vi "Arthur_Q2_VF.vi"() -> ()   [LabVIEW 2019]
uses:
  <vilib>/Waveform/WDTOps.llb/WDT Get Waveform Subset DBL.vi
  <vilib>/measure/matone.llb/Extract Single Tone Information 1 Chan.vi
  <vilib>/measure/NI_MAPro.lvlib
panel:
  out "Numeric 2":dbl
  out "Numeric":dbl
  out "String 2":string="AFUNDAMENTO"
  out "String":string="ELEVA敲O"
  out "Waveform Graph 6":waveform(dbl)(graph)
  out "Waveform Graph 5":waveform(dbl)(graph)
  in  "PATH_2":path=path "C:/lista3.tdms"
  in  "Phase 3":dbl caption="Phase"
  in  "Amplitude 3":dbl=0.5 caption="Amplitude"
  in  "Frequency 3":dbl=40.0 caption="Frequency"
  in  "Phase 2":dbl caption="Phase"
  in  "Amplitude 2":dbl=1.0 caption="Amplitude"
  in  "Frequency 2":dbl=20.0 caption="Frequency"
  in  "Phase":dbl
  in  "Amplitude":dbl=2.0
  in  "Frequency":dbl=10.0
  out "Waveform Graph":dynamicdata(graph)
  # "Phase em graus"
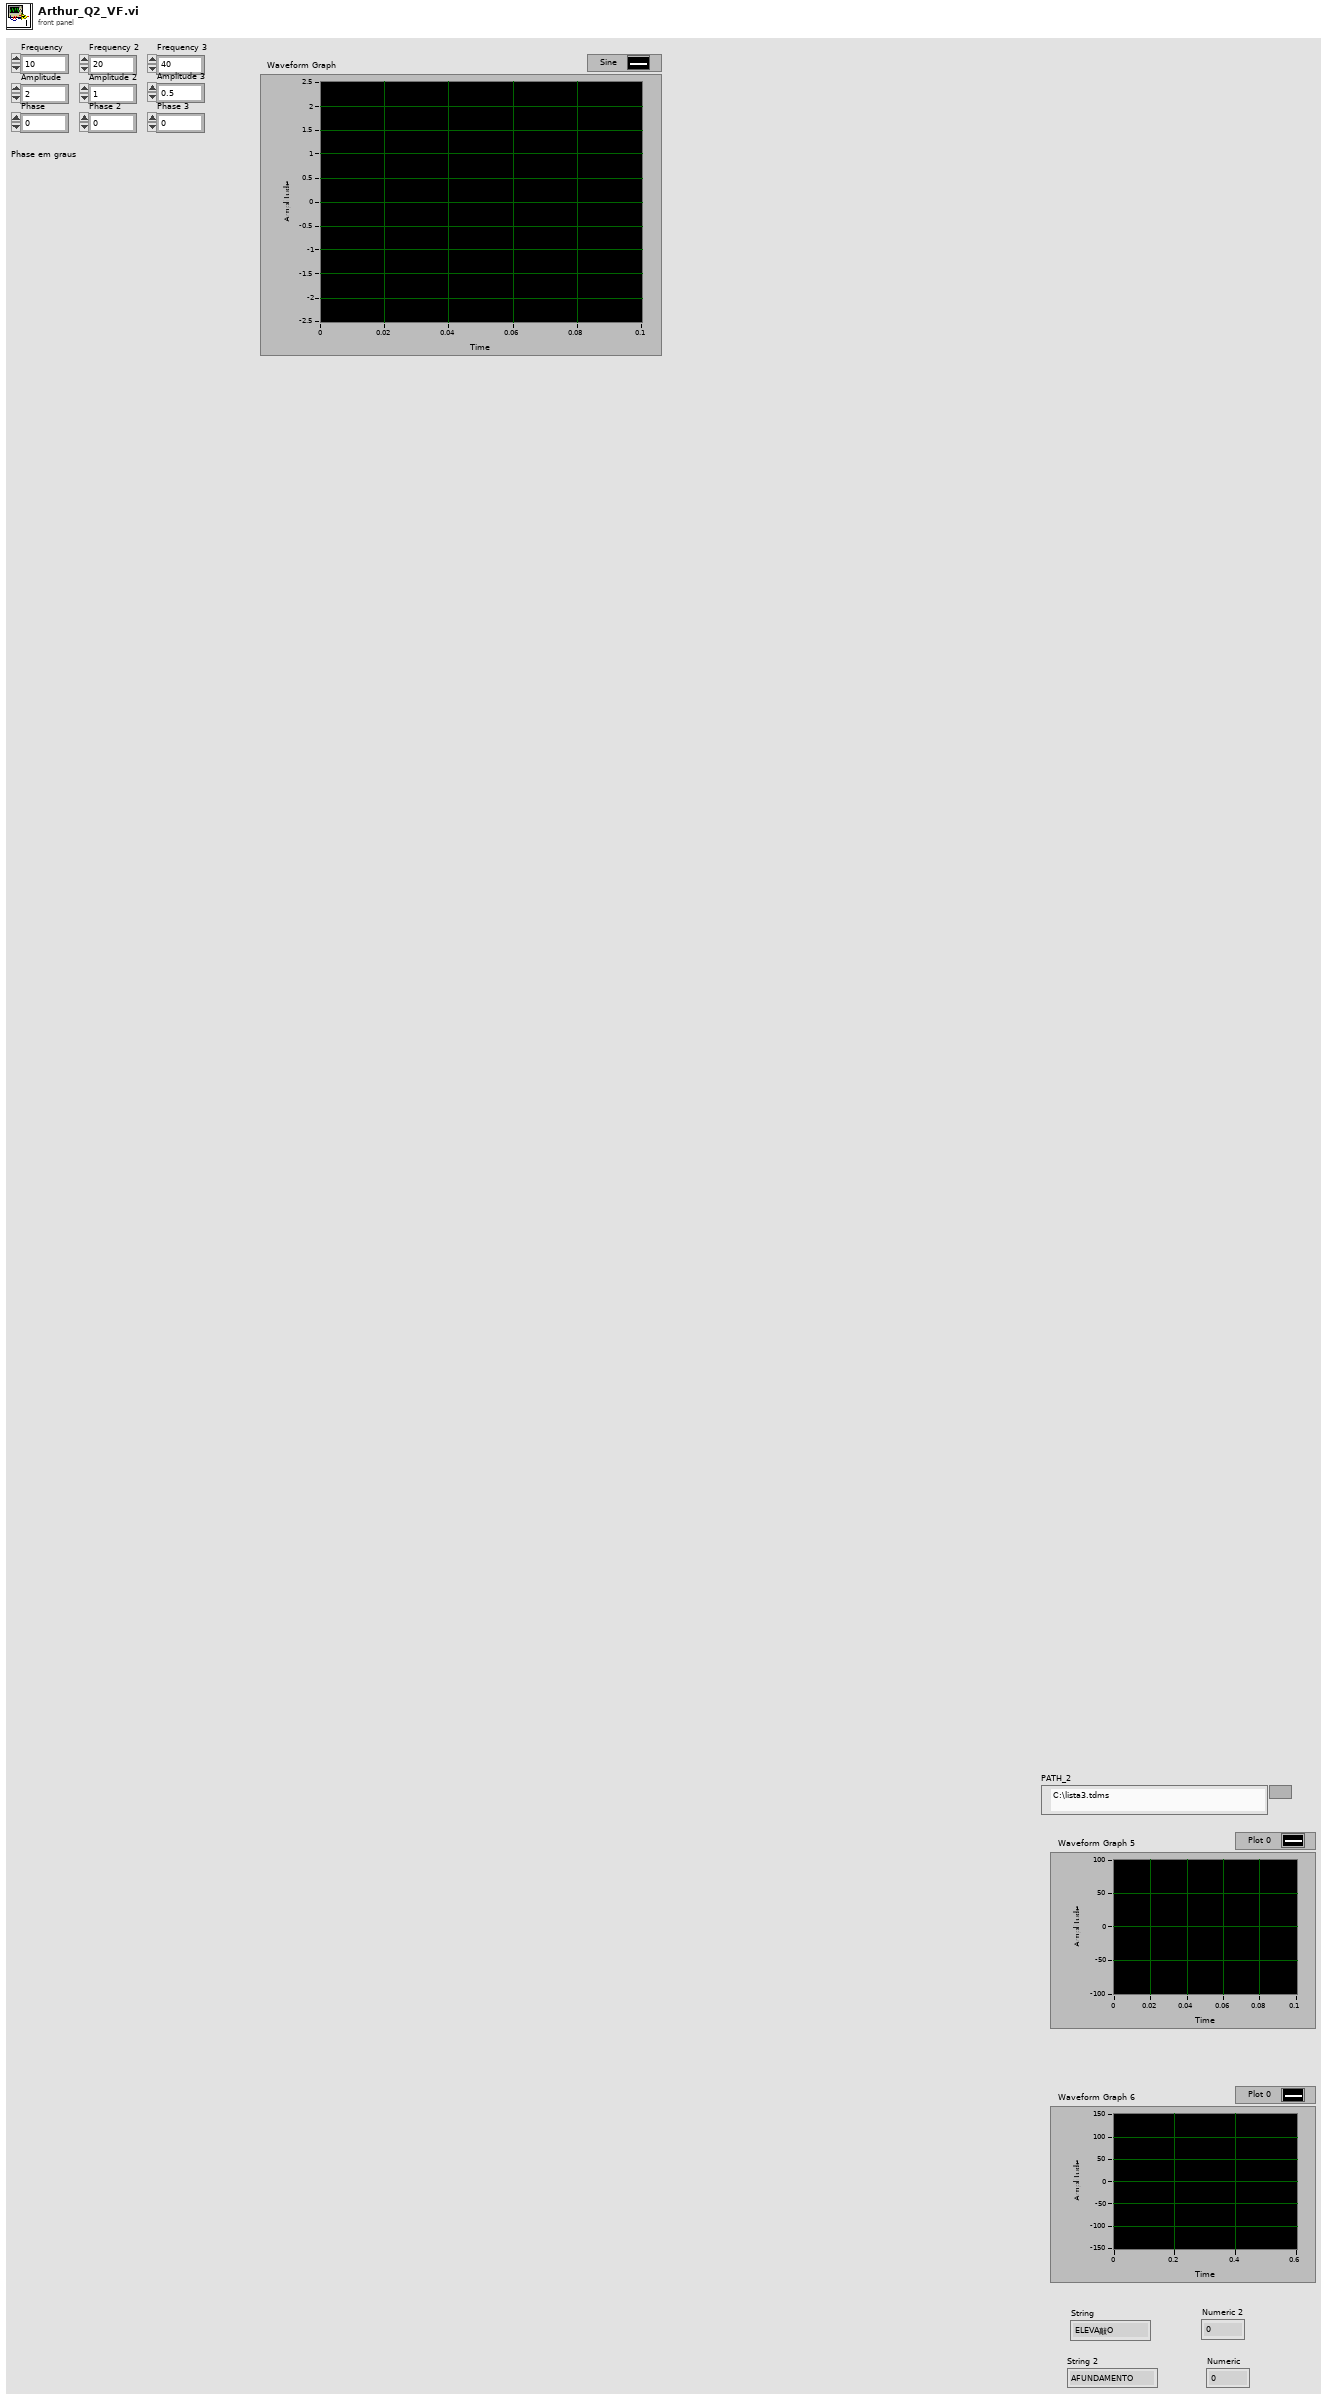
[diagram p1: front panel]
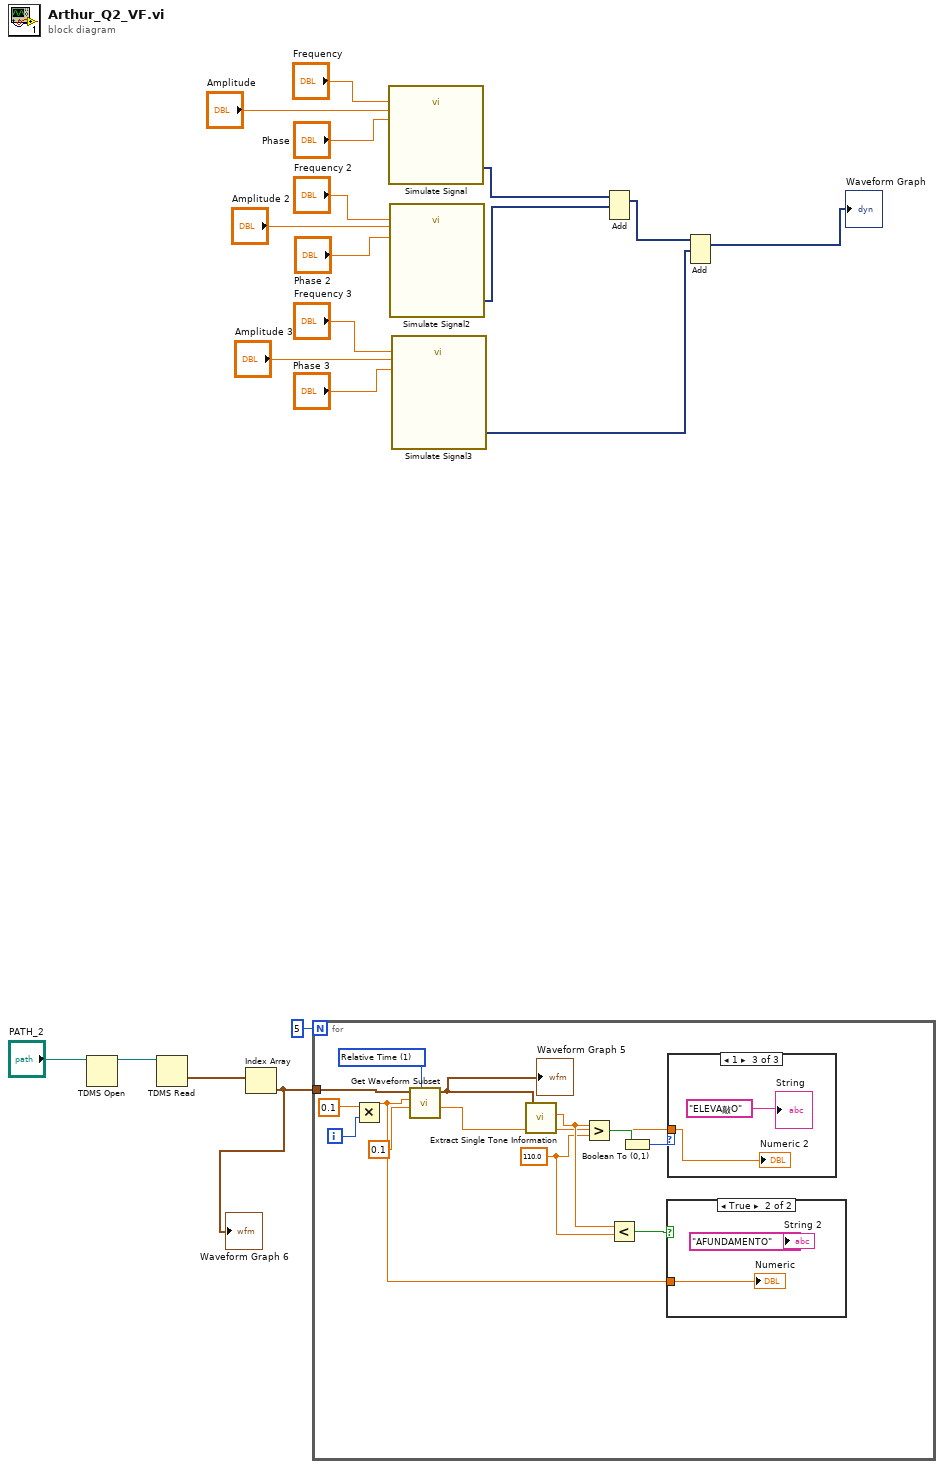
[diagram p0: block diagram]
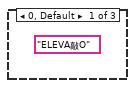
[diagram p3: hidden frame]
diagram:
  n1 = TDMS Open(11:"PATH_2") -> (3:w4:refnum<k34>)  [unwired: 6 in, 1 out]
  n2 = TDMS Read(0:w4) -> (10:w3:waveform(dbl)[])  [unwired: 7 in, 5 out]
  n3 = Index Array(array=w3) -> (element=w2:waveform(dbl))  [unwired: 1 in]
  "Waveform Graph 6" <- w2
  n4 = for {
    N: 5 -> [_]
    tunnel: w2 -> [w32]
    i -> [w30]
    w23 = 110.0 ("y")
    w31 = u16 1 items=["Samples", "Relative Time"] ("start/duration format")
    n5 = Multiply(x=0.1 ("start samples/time"), y=w30) -> (x*y=w21:dbl)
    n6 = call-poly <vilib>:"Get Waveform Subset.vi"("start/duration format"=w31, "duration"=0.1, "start samples/time"=w21, "waveform in"=w32) -> ("actual duration"=w20:dbl, "waveform out"=w27:waveform(dbl))  [unwired: 2 in, 2 out]
    "Waveform Graph 5" <- w27
    n7 = call-poly <vilib>:"Extract Single Tone Information.vi"("time signal in"=w27) -> ("detected amplitude"=w24:dbl)  [unwired: 5 in, 5 out]
    n8 = Greater?(x=w24, y=w23) -> (0:w26:bool)
    n9 = Less?(x=w24, y=w23) -> (x < y?=w22:bool)
    n10 = Boolean To (0,1)(Boolean=w26) -> (0, 1=w25:i16)
    n11 = case shown="True" w22 {
      tunnel: w21 -> [_ w33]
      frame False {
      }
      frame True {
        "String 2" <- "AFUNDAMENTO"
        "Numeric" <- w33
      }
    }
    n12 = case shown="1" w25 {
      tunnel: w20 -> [_ _ w35]
      frame 0, Default {
        (unwired) "ELEVA敲O"
      }
      frame 2 {
      }
      frame 1 {
        "String" <- "ELEVA敲O"
        "Numeric 2" <- w35
      }
    }
  }
  n13 = call "Simulate Signal"("Frequency"="Frequency", "Amplitude"="Amplitude", "Phase"="Phase") -> ("Sine"=w6:dynamicdata)  [unwired: 11 in, 1 out]
  n14 = call "Simulate Signal2"("Frequency"="Frequency 2", "Amplitude"="Amplitude 2", "Phase"="Phase 2") -> ("Sine"=w7:dynamicdata)  [unwired: 11 in, 1 out]
  n15 = call "Simulate Signal3"("Frequency"="Frequency 3", "Amplitude"="Amplitude 3", "Phase"="Phase 3") -> ("Sine"=w9:dynamicdata)  [unwired: 11 in, 1 out]
  n16 = Add(1:w7, 2:w6) -> (0:w8:dynamicdata)  [unwired: 1 in, 1 out]
  n17 = Add(1:w9, 2:w8) -> (0:→"Waveform Graph":dynamicdata)  [unwired: 1 in, 1 out]
